vi "Configure IQ Recorder Measurement Filter.vi"(7 "Bandwidth (100kHz)":dbl=100000.0 format="%#.9p", 8 "error in (no error)":errorcluster, 9 "Filter Type (Gauss)":i32(ring) items=["Gauss", "Bandpass"], 10 "Instance (1)":i32=1 format="%.0g", 11 "VISA resource name":refnum<visa-resource-name>) -> (0 "error out":errorcluster, 3 "VISA resource name out":refnum<visa-resource-name>)   [LabVIEW 2020, in "Rohde&Schwarz CMXP GPRF.lvlib"]
doc: "Configures power measurement filter type and bandwidth.\n\nAttributes:\nRSCMXPGPRF_ATTR_IQ_RECORDER_MEASUREMENT_FILTER_TYPE\nRSCMXPGPRF_ATTR_IQ_RECORDER_MEASUREMENT_GAUSS_BANDWIDTH\nRSCMXPGPRF_ATTR_IQ_RECORDER_MEASUREMENT_BANDPASS_BANDWIDTH\n\nRemote-control commands:\nCONFigure:GPRF:MEAS<i>:IQRecorder:FILTer:TYPE\nCONFigure:GPRF:MEAS<i>:IQRecorder:FILTer:GAUSs:BWIDth\nCONFigure:GPRF:MEAS<i>:IQRecorder:FILTer:BANDpass:BWIDth"
uses:
  <instrlib>/Rohde&Schwarz CMXP GPRF/Rohde&Schwarz CMXP GPRF.lvlib
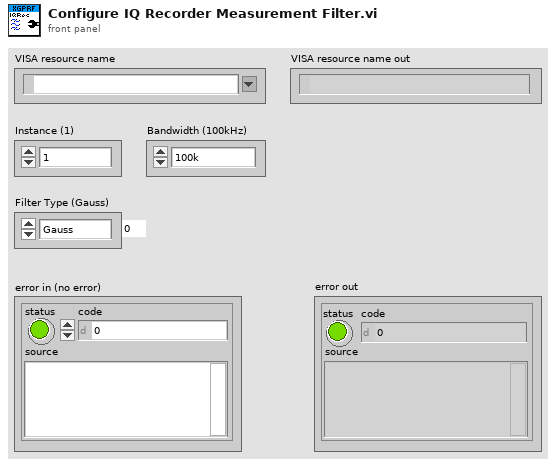
[diagram p1: front panel]
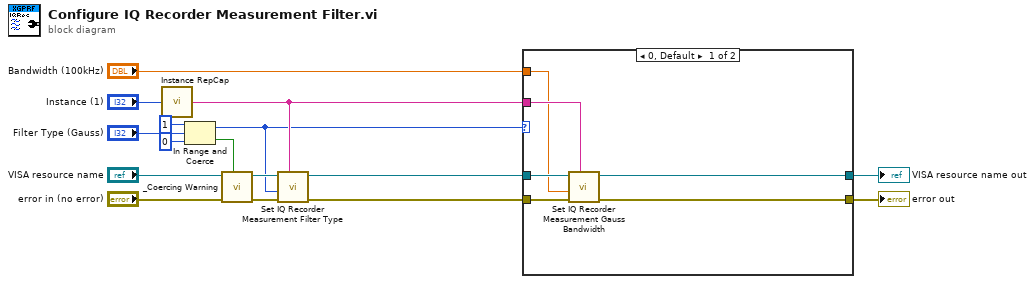
[diagram p0: block diagram]
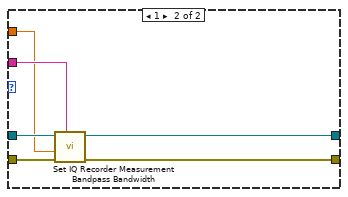
[diagram p2: hidden frame]
diagram:
  n1 = call <instrlib>:"Instance RepCap.vi"("Instance in"="Instance (1)") -> ("Instance out"=w5:string)
  n2 = In Range and Coerce(upper limit=1, x="Filter Type (Gauss)", lower limit=0) -> (coerced(x)=w2:i32, In Range?=w10:bool)
  n3 = call <instrlib>:"_Coercing Warning.vi"("In Range?"=w10, "error in (no error)"="error in (no error)", "VISA resource name"="VISA resource name") -> ("error out"=w11:errorcluster, "VISA resource name out"=w12:refnum<visa-resource-name>)  [unwired: 7 in]
  n4 = call "Set IQ Recorder Measurement Filter Type"("Repeated Capabilities"=w5, "error in (no error)"=w11, "IQ Recorder Measurement Filter Type (0 - Gauss)"=w2, "instrument handle"=w12) -> ("error out"=w15:errorcluster, "instrument handle out"=w16:refnum<visa-resource-name>)  [unwired: 6 in]
  n5 = case shown="0, Default" w2 {
    tunnel: w16 -> [w22 w28]
    tunnel: w15 -> [w21 w27]
    tunnel: "Bandwidth (100kHz)" -> [w17 w23]
    tunnel: [w18 w24] -> w8
    tunnel: [w19 w25] -> w7
    tunnel: w5 -> [w20 w26]
    frame 0, Default {
      n6 = call "Set IQ Recorder Measurement Gauss Bandwidth"("Repeated Capabilities"=w20, "error in (no error)"=w21, "IQ Recorder Measurement Gauss Bandwidth (0.0)"=w17, "instrument handle"=w22) -> ("error out"=w19:errorcluster, "instrument handle out"=w18:refnum<visa-resource-name>)  [unwired: 6 in]
    }
    frame 1 {
      n7 = call "Set IQ Recorder Measurement Bandpass Bandwidth"("Repeated Capabilities"=w26, "error in (no error)"=w27, "IQ Recorder Measurement Bandpass Bandwidth (0.0)"=w23, "instrument handle"=w28) -> ("error out"=w25:errorcluster, "instrument handle out"=w24:refnum<visa-resource-name>)  [unwired: 6 in]
    }
  }
  "error out" <- w7
  "VISA resource name out" <- w8
